vi "Limit Testing Measurement.vi"() -> ()   [LabVIEW 2023]
doc: "This example creates limit waveforms and performs limit testing on the test signal. The test signal is a combination of a square waveform and a uniform white noise waveform. Upper Limit and Lower Limit specify the X and the Y axis values for the upper and lower limit. You input the test waveform and the limit waveforms to the Limit Testing VI. You can wire the output of this VI to a waveform graph."
uses:
  <vilib>/measure/mamon.llb/Limit Specification.vi
  <vilib>/measure/mamon.llb/Limit Testing Time.vi
  <vilib>/measure/NI_MAPro.lvlib
  <vilib>/measure/NI_MABase.lvlib
panel:
  in  "Noise":dbl(slide)=0.08080808080808081 scale=0.0..1.0
  in  "Lower Limit":cluster{"X values":dbl[], "Y values":dbl[]}={"X values"=[0.0, 0.45, 0.46, 1.05, 1.06, 1.45, 1.46, 2.05, 2.06, 2.45, 2.46], "Y values"=[0.9, 0.9, -1.1, -1.1, 0.9, 0.9, -1.1, -1.1, 0.9, 0.9, -1.1]}
  in  "Upper Limit":cluster{"X values":dbl[], "Y values":dbl[]}={"X values"=[0.0, 0.54, 0.55, 0.99, 1.0, 1.54, 1.55, 1.99, 2.0, 2.49, 2.5], "Y values"=[1.1, 1.1, -0.9, -0.9, 1.1, 1.1, -0.9, -0.9, 1.1, 1.1, -0.9]}
  out "test passed?":bool
  in  "Stop":bool
  out "Limit Test":waveform(dbl)[](graph)
  # "Overview: This example creates limit waveforms and performs limit testing on the test signal.  \nRequirements: LabVIEW Full Development System\nInstructions: \n1. Run the VI. Note that the limit test passes - the signal fits within the Upper Limit and Lower Limit.\n2. Increase the Noise, and note that the limit test fails when the signal is outside of the limit bounds.\n3. Click Stop to stop the VI."
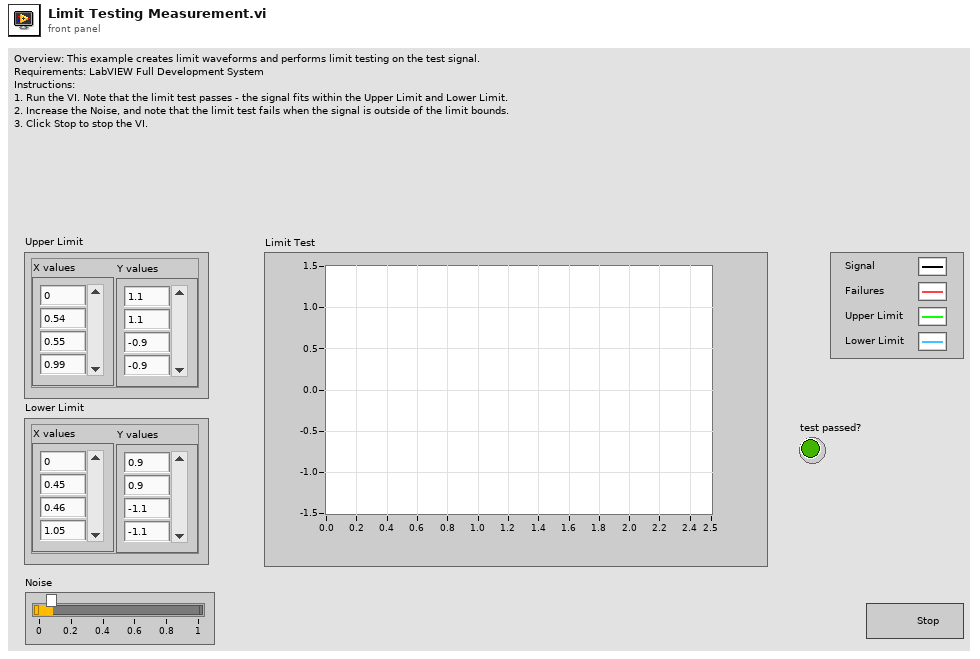
[diagram p1: front panel]
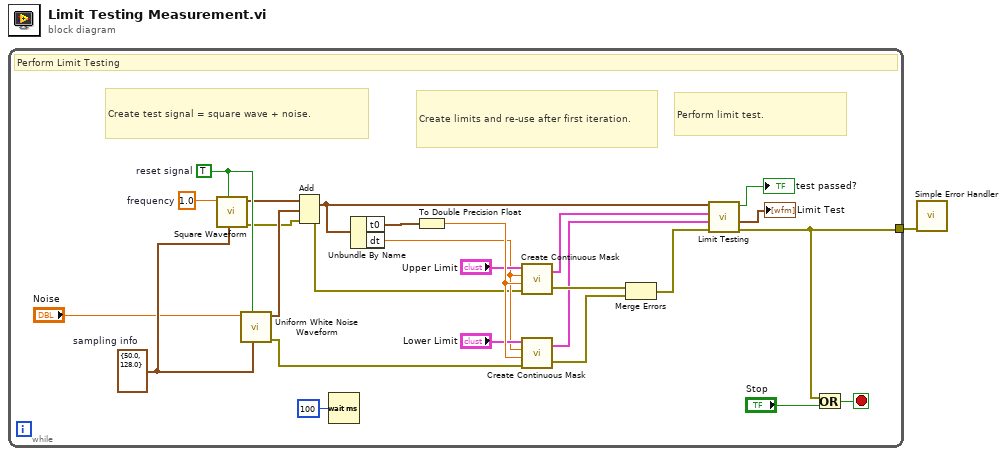
[diagram p0: block diagram]
diagram:
  n1 = while {
    tunnel: [w7] -> w1
    stop <- w10 stop-if-true
    w2 = 1.0  # frequency
    w12 = TRUE  # reset signal
    w25 = cluster{"Fs":dbl, "#s":dbl} {"Fs"=50.0, "#s"=128.0}  # sampling info
    # "Create test signal = square wave + noise."
    # "Perform limit test."
    # "Create limits and re-use after first iteration."
    # "Perform Limit Testing"
    n2 = call <vilib>:"Square Waveform.vi"("sampling info"=w25, "reset signal"=w12, "frequency"=w2) -> ("error out"=w4:errorcluster, "signal out"=w8:waveform(dbl))  [unwired: 7 in]
    n3 = call <vilib>:"Uniform White Noise Waveform.vi"("sampling info"=w25, "reset signal"=w12, "amplitude"="Noise") -> ("error out"=w5:errorcluster, "signal out"=w18:waveform(dbl))  [unwired: 7 in]
    n4 = Add(1:w18, 2:w8, 4:w4) -> (0:w17:waveform(dbl), 3:w3:errorcluster)
    n5 = Wait (ms)(milliseconds to wait=u32 100) -> ()  [unwired: 1 out]
    n6 = Unbundle By Name(w17) -> ("t0"=w15:timestamp, "dt"=w9:dbl)
    n7 = To Double Precision Float(number=w15) -> (double precision float=w19:dbl)
    n8 = call-poly <vilib>:"Create Continuous Mask.vi"("Specification Cluster"="Upper Limit", "dx"=w9, "x0"=w19, "error in (no error)"=w3) -> ("Limit"=w20:cluster{"x0":dbl, "dx":dbl, "Y":dbl[]}, "error out"=w23:errorcluster)  [unwired: 1 in]
    n9 = call-poly <vilib>:"Create Continuous Mask.vi"("Specification Cluster"="Lower Limit", "dx"=w9, "x0"=w19, "error in (no error)"=w5) -> ("Limit"=w6:cluster{"x0":dbl, "dx":dbl, "Y":dbl[]}, "error out"=w22:errorcluster)  [unwired: 1 in]
    n10 = Merge Errors(w23, w22) -> (w21:errorcluster)
    n11 = call-poly <vilib>:"Limit Testing.vi"("error in (no error)"=w21, "lower limit"=w6, "upper limit"=w20, "signal in"=w17) -> ("error out"=w7:errorcluster, "output values"=→"Limit Test":waveform(dbl)[], "test passed?"=→"test passed?":bool)  [unwired: 2 in, 3 out]
    n12 = Or(x=w7, y="Stop") -> (x .or. y?=w10:bool)
  }
  n13 = call <vilib>:"Simple Error Handler.vi"("error in (no error)"=w1) -> ()  [unwired: 4 in, 5 out]
